vi "Transmitter HMI Main.vi"() -> ()   [LabVIEW 2025]
uses:
  Globals/Cancelled Global.vi
  Globals/Percent Complete Global.vi
  Globals/Light VISA Global.vi
  <vilib>/Instr/_visa.llb/VISA Configure Serial Port (Instr).vi
  Globals/Solenoid VISA Global.vi
  Globals/Touch VISA Global.vi
  Globals/Motor VISA Global.vi
  Globals/Wire VISA Global.vi
  Globals/QRCode VISA Global.vi
panel:
  in  "Enable Wire":bool
  in  "Enable Barcode":bool
  in  "Enable Motor":bool
  in  "Enable Light":bool
  in  "Enable Touch":bool
  in  "Enable Solenoid":bool
  in  "FREQUENCY CHANGER":bool
  in  "Barcode":bool
  in  "Wire":bool
  out "Start Transmission":bool
  out "Exit":bool
  out "Transmitting":bool
  out "Chosen Text":string
  out "Chosen Image Path":path caption="selected path"
  out "Chosen Transmission Method":u16(ring) items=["Barcode", "Wire", "Motor", "Touch", "Light", "Solenoid"]
  out "Chosen Data Type":u16(ring) items=["Text File", "Image File", "Image", "Text"]
  in  "Cancel Button":bool
  out "Transmission Progress:":dbl(slide) scale=0.0..100.0
  in  "Go":bool
  in  "Motor":bool
  in  "Touch":bool
  in  "Light":bool
  in  "Solenoid":bool
  in  "Image":bool
  in  "Text":bool
  # "TRANSMITTER"
  # "1: Select Data Type:"
  # "2: Select Method of Transmission:"
  # "3: BEGIN"
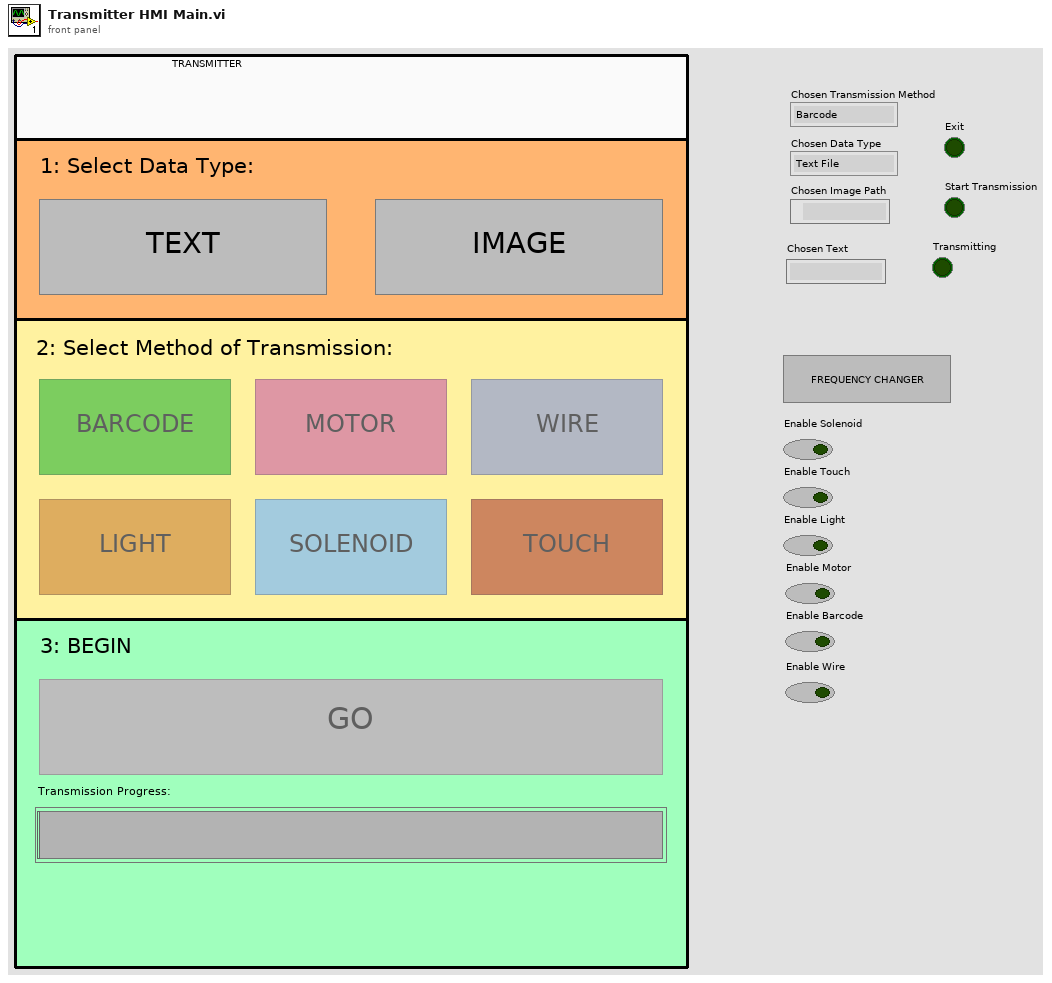
[diagram p1: front panel]
types:
  T1 = enum8{"Enabled", "Disabled", "Disabled and Grayed Out"}
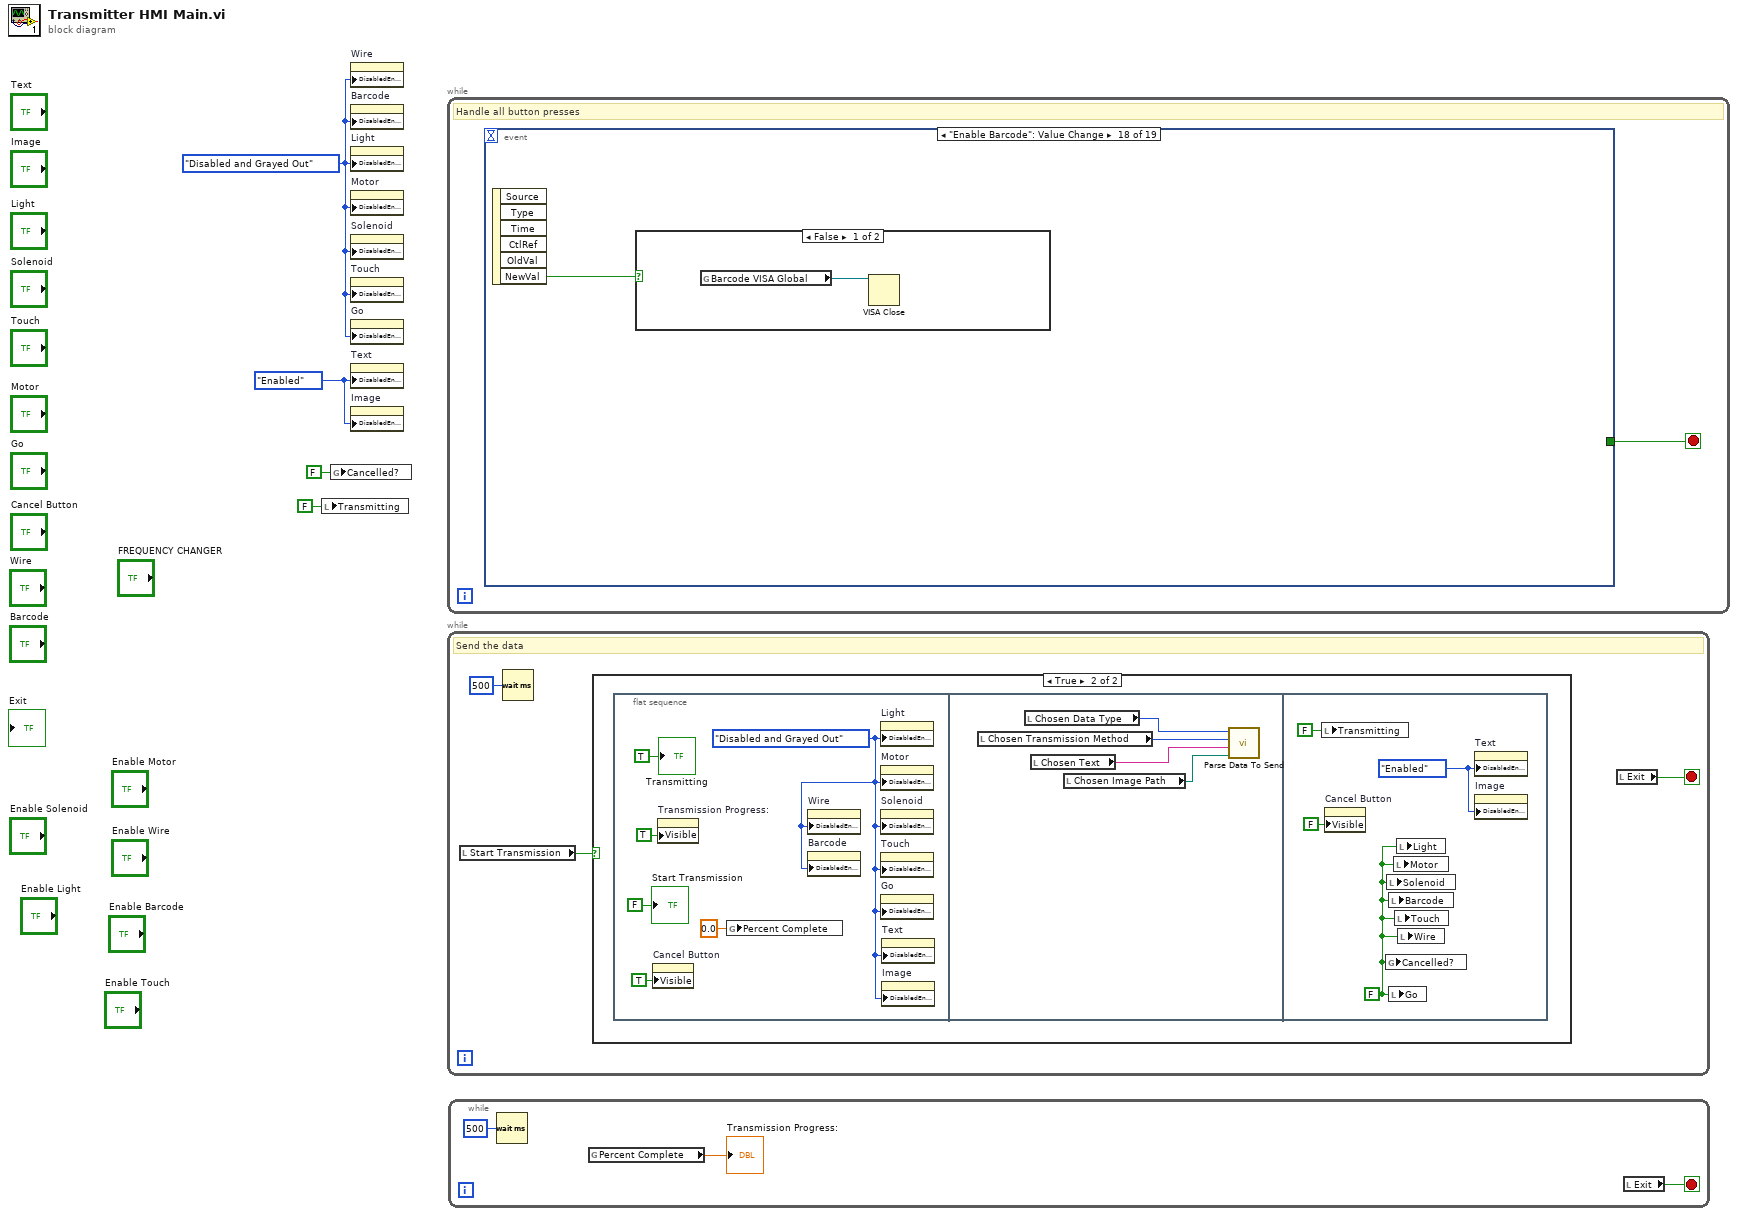
[diagram p0: block diagram]
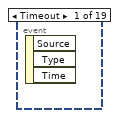
[diagram p3: hidden frame]
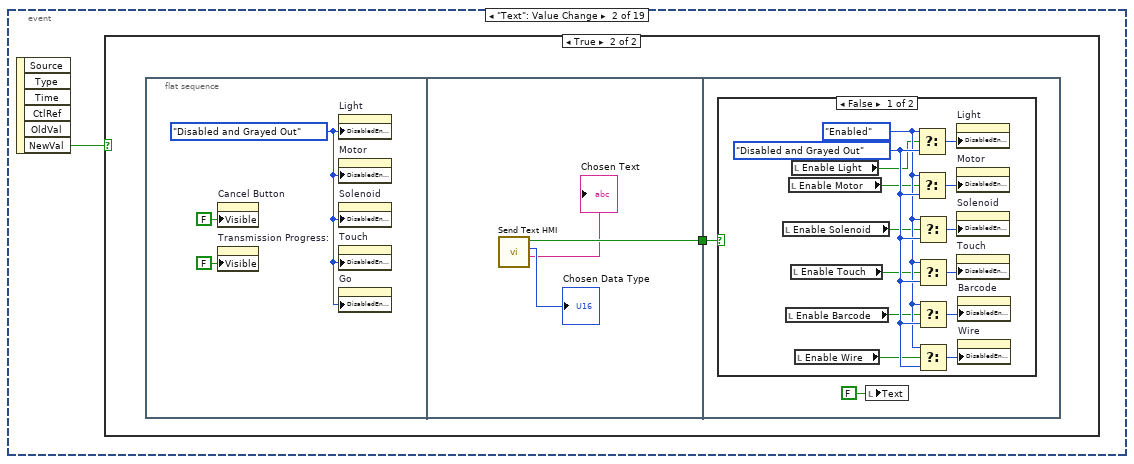
[diagram p4: hidden frame]
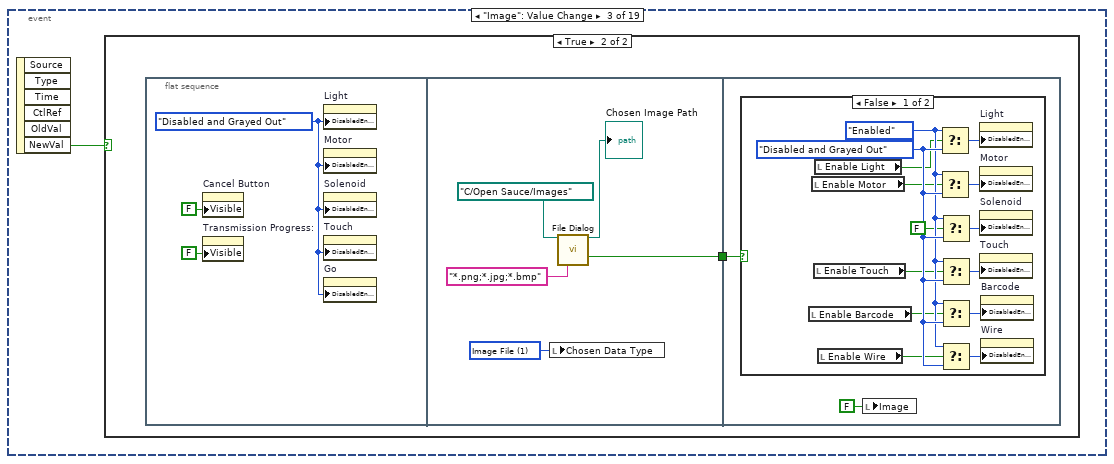
[diagram p7: hidden frame]
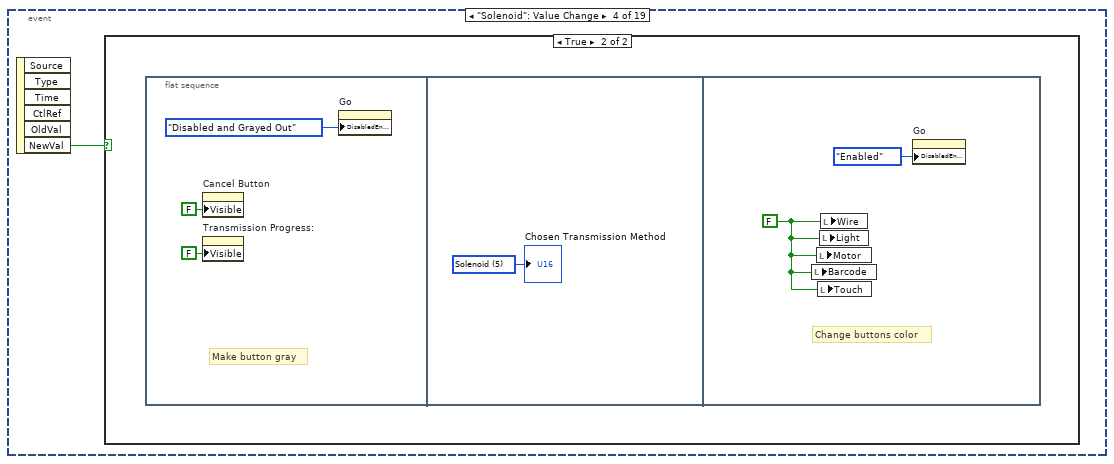
[diagram p10: hidden frame]
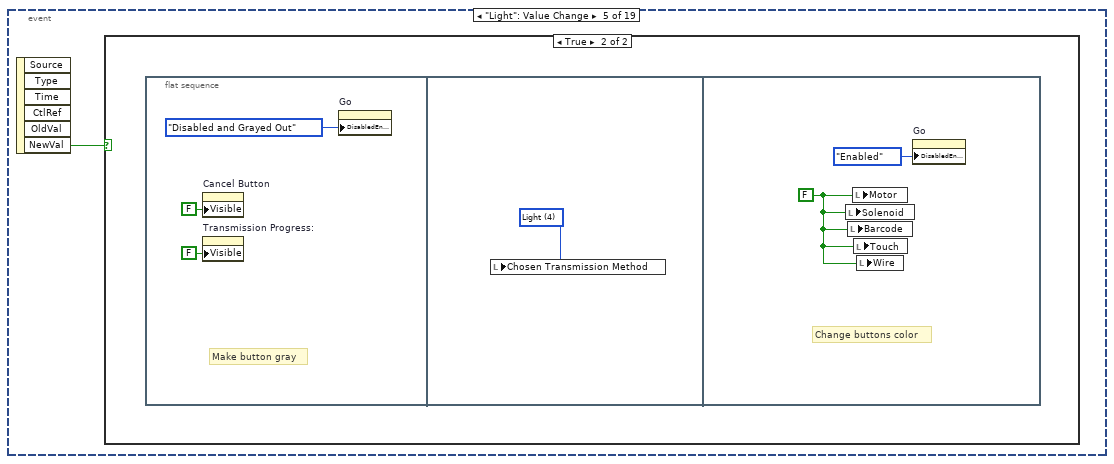
[diagram p12: hidden frame]
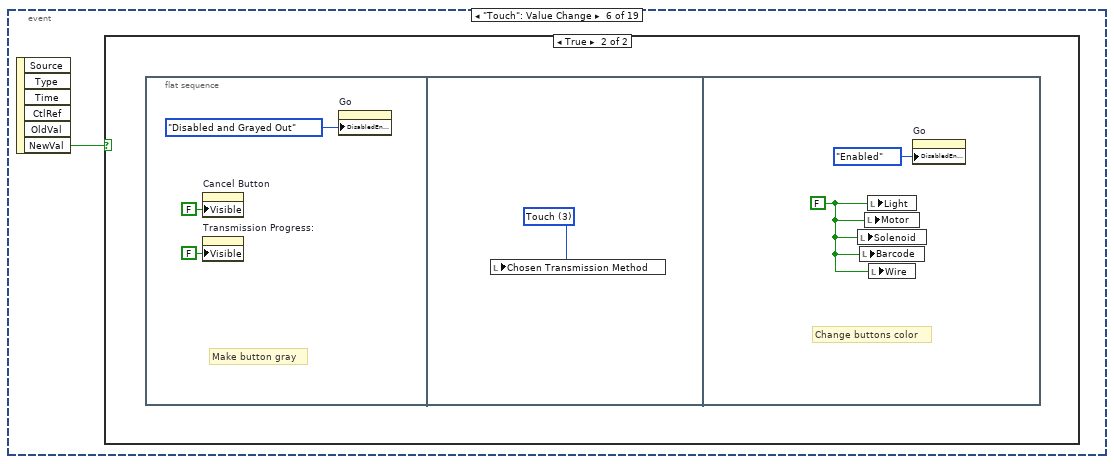
[diagram p14: hidden frame]
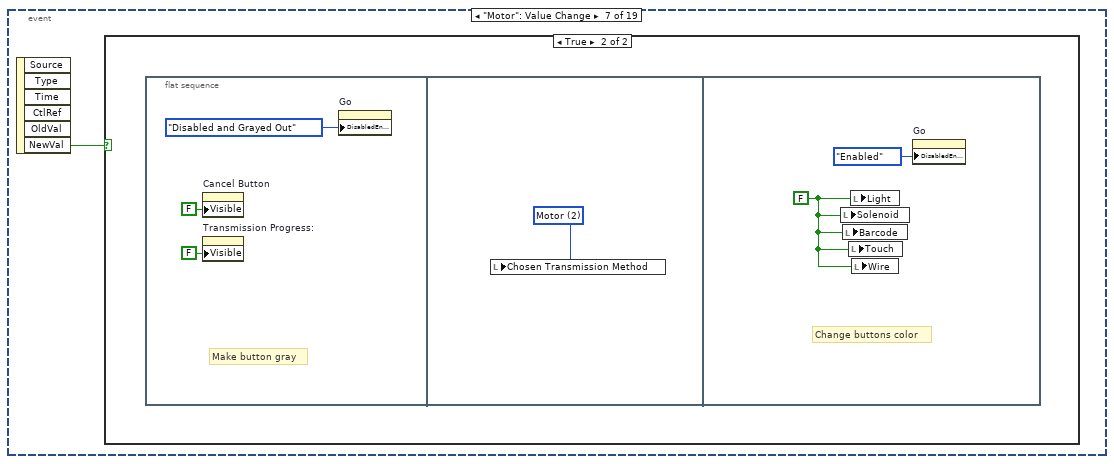
[diagram p16: hidden frame]
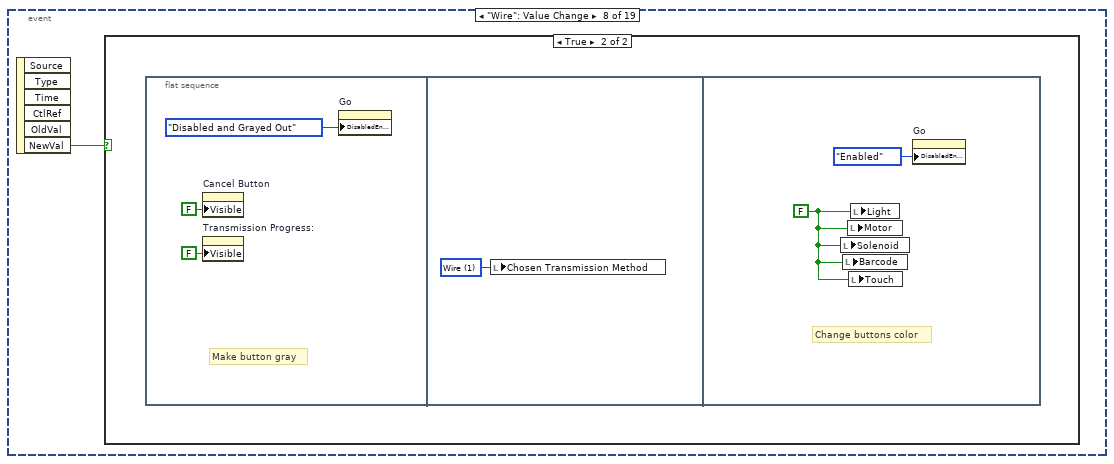
[diagram p18: hidden frame]
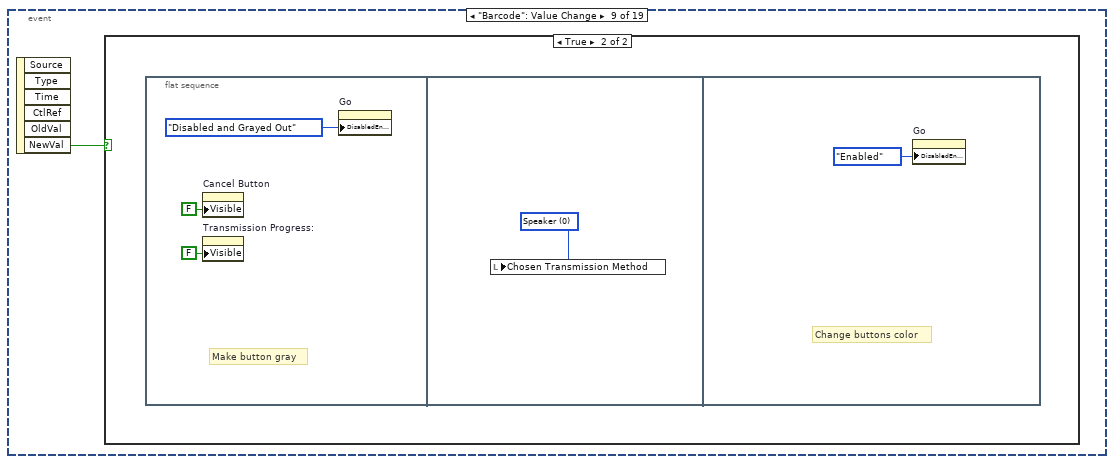
[diagram p20: hidden frame]
diagram:
  w2 = T1."Enabled" ("Disabled")
  w1 = T1."Disabled and Grayed Out" ("Disabled")
  n1 = local write "Transmitting"(FALSE ("Transmitting")) -> ()
  n2 = global write "Cancelled Global.vi" "Cancelled?"(FALSE ("Cancelled?")) -> ()
  n3 = property on="Wire" class="Bool (strict)"("DisabledEnum"=w1) -> ()  [unwired: 2 in, 2 out]
  n4 = property on="Barcode" class="Bool (strict)"("DisabledEnum"=w1) -> ()  [unwired: 2 in, 2 out]
  n5 = property on="Light" class="Bool (strict)"("DisabledEnum"=w1) -> ()  [unwired: 2 in, 2 out]
  n6 = property on="Motor" class="Bool (strict)"("DisabledEnum"=w1) -> ()  [unwired: 2 in, 2 out]
  n7 = property on="Solenoid" class="Bool (strict)"("DisabledEnum"=w1) -> ()  [unwired: 2 in, 2 out]
  n8 = property on="Touch" class="Bool (strict)"("DisabledEnum"=w1) -> ()  [unwired: 2 in, 2 out]
  n9 = property on="Go" class="Bool (strict)"("DisabledEnum"=w1) -> ()  [unwired: 2 in, 2 out]
  n10 = property on="Text" class="Bool (strict)"("DisabledEnum"=w2) -> ()  [unwired: 2 in, 2 out]
  n11 = property on="Image" class="Bool (strict)"("DisabledEnum"=w2) -> ()  [unwired: 2 in, 2 out]
  n12 = while {
    stop <- w5 stop-if-true
    # "Handle all button presses"
    n13 = event shown="[17] \"Enable Barcode\": Value Change" {
      selector: _ -> [_ _ _ _ _ _ _ _ _ _ _ _ _ _ _ _ _ _ _]
      dyn-events: _ -> [_ _ _ _ _ _ _ _ _ _ _ _ _ _ _ _ _ _ _]
      timeout: _ -> [_ _ _ _ _ _ _ _ _ _ _ _ _ _ _ _ _ _ _]
      tunnel: [_ _ _ _ _ _ _ _ _ TRUE _ _ _ _ _ _ _ _ _] -> w5
      event Timeout {
        n14 = event-data() -> ()  [unwired: 1 in, 3 out]
      }
      event "Text": Value Change {
        n15 = event-data() -> ("NewVal"=w6:bool)  [unwired: 1 in, 5 out]
        n16 = case shown="True" w6 {
          frame False {
          }
          frame True {
            n17 = flat-sequence {
              tunnel: [w13] -> w7
              tunnel: w7 -> [w15]
              frame #0 {
                w9 = T1."Disabled and Grayed Out" ("Disabled")
                n18 = property on="Cancel Button" class="Bool (strict)"("Visible"=FALSE) -> ()  [unwired: 2 in, 2 out]
                n19 = property on="Transmission Progress:" class="Slide (strict)"("Visible"=FALSE) -> ()  [unwired: 2 in, 2 out]
                n20 = property on="Light" class="Bool (strict)"("DisabledEnum"=w9) -> ()  [unwired: 2 in, 2 out]
                n21 = property on="Motor" class="Bool (strict)"("DisabledEnum"=w9) -> ()  [unwired: 2 in, 2 out]
                n22 = property on="Solenoid" class="Bool (strict)"("DisabledEnum"=w9) -> ()  [unwired: 2 in, 2 out]
                n23 = property on="Touch" class="Bool (strict)"("DisabledEnum"=w9) -> ()  [unwired: 2 in, 2 out]
                n24 = property on="Go" class="Bool (strict)"("DisabledEnum"=w9) -> ()  [unwired: 2 in, 2 out]
              }
              frame #1 {
                n25 = call "Send Text HMI.vi"() -> ("Chosen Text"=→"Chosen Text":string, "Chosen Data Type"=→"Chosen Data Type":u16, "Cancelled"=w13:bool)  [unwired: 9 in]
              }
              frame #2 {
                n26 = case shown="False" w15 {
                  frame False {
                    w23 = T1."Disabled and Grayed Out" ("Disabled")
                    w22 = T1."Enabled" ("Disabled")
                    n27 = local read "Enable Solenoid"() -> (w18:bool)
                    n28 = local read "Enable Barcode"() -> (w20:bool)
                    n29 = local read "Enable Motor"() -> (w17:bool)
                    n30 = local read "Enable Touch"() -> (w19:bool)
                    n31 = local read "Enable Light"() -> (w16:bool)
                    n32 = local read "Enable Wire"() -> (w21:bool)
                    n33 = Select(t=w22, s=w16, f=w23) -> (s? t:f=w29:T1)
                    n34 = Select(t=w22, s=w17, f=w23) -> (s? t:f=w28:T1)
                    n35 = Select(t=w22, s=w18, f=w23) -> (s? t:f=w27:T1)
                    n36 = Select(t=w22, s=w19, f=w23) -> (s? t:f=w26:T1)
                    n37 = Select(t=w22, s=w20, f=w23) -> (s? t:f=w25:T1)
                    n38 = Select(t=w22, s=w21, f=w23) -> (s? t:f=w24:T1)
                    n39 = property on="Light" class="Bool (strict)"("DisabledEnum"=w29) -> ()  [unwired: 2 in, 2 out]
                    n40 = property on="Motor" class="Bool (strict)"("DisabledEnum"=w28) -> ()  [unwired: 2 in, 2 out]
                    n41 = property on="Solenoid" class="Bool (strict)"("DisabledEnum"=w27) -> ()  [unwired: 2 in, 2 out]
                    n42 = property on="Touch" class="Bool (strict)"("DisabledEnum"=w26) -> ()  [unwired: 2 in, 2 out]
                    n43 = property on="Barcode" class="Bool (strict)"("DisabledEnum"=w25) -> ()  [unwired: 2 in, 2 out]
                    n44 = property on="Wire" class="Bool (strict)"("DisabledEnum"=w24) -> ()  [unwired: 2 in, 2 out]
                  }
                  frame True {
                  }
                }
                n45 = local write "Text"(FALSE ("Text")) -> ()
              }
            }
          }
        }
      }
      event "Image": Value Change {
        n46 = event-data() -> ("NewVal"=w30:bool)  [unwired: 1 in, 5 out]
        n47 = case shown="True" w30 {
          frame False {
          }
          frame True {
            n48 = flat-sequence {
              tunnel: [w37] -> w31
              tunnel: w31 -> [w40]
              frame #0 {
                w33 = T1."Disabled and Grayed Out" ("Disabled")
                n49 = property on="Cancel Button" class="Bool (strict)"("Visible"=FALSE) -> ()  [unwired: 2 in, 2 out]
                n50 = property on="Transmission Progress:" class="Slide (strict)"("Visible"=FALSE) -> ()  [unwired: 2 in, 2 out]
                n51 = property on="Light" class="Bool (strict)"("DisabledEnum"=w33) -> ()  [unwired: 2 in, 2 out]
                n52 = property on="Motor" class="Bool (strict)"("DisabledEnum"=w33) -> ()  [unwired: 2 in, 2 out]
                n53 = property on="Solenoid" class="Bool (strict)"("DisabledEnum"=w33) -> ()  [unwired: 2 in, 2 out]
                n54 = property on="Touch" class="Bool (strict)"("DisabledEnum"=w33) -> ()  [unwired: 2 in, 2 out]
                n55 = property on="Go" class="Bool (strict)"("DisabledEnum"=w33) -> ()  [unwired: 2 in, 2 out]
              }
              frame #1 {
                w35 = u16 1 items=["Text File", "Image File", "Image", "Text"] ("Chosen Data Type")
                n56 = local write "Chosen Data Type"(w35) -> ()
                n57 = call "File Dialog"("start path"=path "C:/Open Sauce/Images", "pattern (all files)"="*.png;*.jpg;*.bmp") -> ("selected path"=→"Chosen Image Path":path, "cancelled"=w37:bool)  [unwired: 10 in, 2 out]
              }
              frame #2 {
                n58 = case shown="False" w40 {
                  frame False {
                    w49 = T1."Disabled and Grayed Out" ("Disabled")
                    w48 = T1."Enabled" ("Disabled")
                    n59 = local read "Enable Barcode"() -> (w46:bool)
                    n60 = local read "Enable Motor"() -> (w44:bool)
                    n61 = local read "Enable Touch"() -> (w45:bool)
                    n62 = local read "Enable Light"() -> (w43:bool)
                    n63 = local read "Enable Wire"() -> (w47:bool)
                    n64 = Select(t=w48, s=w43, f=w49) -> (s? t:f=w55:T1)
                    n65 = Select(t=w48, s=w44, f=w49) -> (s? t:f=w54:T1)
                    n66 = Select(t=w48, s=FALSE, f=w49) -> (s? t:f=w53:T1)
                    n67 = Select(t=w48, s=w45, f=w49) -> (s? t:f=w52:T1)
                    n68 = Select(t=w48, s=w46, f=w49) -> (s? t:f=w51:T1)
                    n69 = Select(t=w48, s=w47, f=w49) -> (s? t:f=w50:T1)
                    n70 = property on="Light" class="Bool (strict)"("DisabledEnum"=w55) -> ()  [unwired: 2 in, 2 out]
                    n71 = property on="Motor" class="Bool (strict)"("DisabledEnum"=w54) -> ()  [unwired: 2 in, 2 out]
                    n72 = property on="Solenoid" class="Bool (strict)"("DisabledEnum"=w53) -> ()  [unwired: 2 in, 2 out]
                    n73 = property on="Touch" class="Bool (strict)"("DisabledEnum"=w52) -> ()  [unwired: 2 in, 2 out]
                    n74 = property on="Barcode" class="Bool (strict)"("DisabledEnum"=w51) -> ()  [unwired: 2 in, 2 out]
                    n75 = property on="Wire" class="Bool (strict)"("DisabledEnum"=w50) -> ()  [unwired: 2 in, 2 out]
                  }
                  frame True {
                  }
                }
                n76 = local write "Image"(FALSE ("Text")) -> ()
              }
            }
          }
        }
      }
      event "Solenoid": Value Change {
        n77 = event-data() -> ("NewVal"=w56:bool)  [unwired: 1 in, 5 out]
        n78 = case shown="True" w56 {
          frame False {
          }
          frame True {
            n79 = flat-sequence {
              frame #0 {
                # "Make button gray"
                n80 = property on="Cancel Button" class="Bool (strict)"("Visible"=FALSE) -> ()  [unwired: 2 in, 2 out]
                n81 = property on="Transmission Progress:" class="Slide (strict)"("Visible"=FALSE) -> ()  [unwired: 2 in, 2 out]
                n82 = property on="Go" class="Bool (strict)"("DisabledEnum"=T1."Disabled and Grayed Out" ("Disabled")) -> ()  [unwired: 2 in, 2 out]
              }
              frame #1 {
                w60 = u16 5 items=["Speaker", "Wire", "Motor", "Touch", "Light", "Solenoid"] ("Chosen Transmission Method")
                "Chosen Transmission Method" <- w60
              }
              frame #2 {
                w61 = FALSE ("Text")
                # "Change buttons color"
                n83 = local write "Barcode"(w61) -> ()
                n84 = local write "Motor"(w61) -> ()
                n85 = local write "Touch"(w61) -> ()
                n86 = local write "Light"(w61) -> ()
                n87 = local write "Wire"(w61) -> ()
                n88 = property on="Go" class="Bool (strict)"("DisabledEnum"=T1."Enabled" ("Disabled")) -> ()  [unwired: 2 in, 2 out]
              }
            }
          }
        }
      }
      event "Light": Value Change {
        n89 = event-data() -> ("NewVal"=w63:bool)  [unwired: 1 in, 5 out]
        n90 = case shown="True" w63 {
          frame False {
          }
          frame True {
            n91 = flat-sequence {
              frame #0 {
                # "Make button gray"
                n92 = property on="Cancel Button" class="Bool (strict)"("Visible"=FALSE) -> ()  [unwired: 2 in, 2 out]
                n93 = property on="Transmission Progress:" class="Slide (strict)"("Visible"=FALSE) -> ()  [unwired: 2 in, 2 out]
                n94 = property on="Go" class="Bool (strict)"("DisabledEnum"=T1."Disabled and Grayed Out" ("Disabled")) -> ()  [unwired: 2 in, 2 out]
              }
              frame #1 {
                w67 = u16 4 items=["Speaker", "Wire", "Motor", "Touch", "Light", "Solenoid"] ("Chosen Transmission Method")
                n95 = local write "Chosen Transmission Method"(w67) -> ()
              }
              frame #2 {
                w68 = FALSE ("Text")
                # "Change buttons color"
                n96 = local write "Solenoid"(w68) -> ()
                n97 = local write "Barcode"(w68) -> ()
                n98 = local write "Motor"(w68) -> ()
                n99 = local write "Touch"(w68) -> ()
                n100 = local write "Wire"(w68) -> ()
                n101 = property on="Go" class="Bool (strict)"("DisabledEnum"=T1."Enabled" ("Disabled")) -> ()  [unwired: 2 in, 2 out]
              }
            }
          }
        }
      }
      event "Touch": Value Change {
        n102 = event-data() -> ("NewVal"=w70:bool)  [unwired: 1 in, 5 out]
        n103 = case shown="True" w70 {
          frame False {
          }
          frame True {
            n104 = flat-sequence {
              frame #0 {
                # "Make button gray"
                n105 = property on="Cancel Button" class="Bool (strict)"("Visible"=FALSE) -> ()  [unwired: 2 in, 2 out]
                n106 = property on="Transmission Progress:" class="Slide (strict)"("Visible"=FALSE) -> ()  [unwired: 2 in, 2 out]
                n107 = property on="Go" class="Bool (strict)"("DisabledEnum"=T1."Disabled and Grayed Out" ("Disabled")) -> ()  [unwired: 2 in, 2 out]
              }
              frame #1 {
                w74 = u16 3 items=["Speaker", "Wire", "Motor", "Touch", "Light", "Solenoid"] ("Chosen Transmission Method")
                n108 = local write "Chosen Transmission Method"(w74) -> ()
              }
              frame #2 {
                w75 = FALSE ("Text")
                # "Change buttons color"
                n109 = local write "Solenoid"(w75) -> ()
                n110 = local write "Barcode"(w75) -> ()
                n111 = local write "Motor"(w75) -> ()
                n112 = local write "Light"(w75) -> ()
                n113 = local write "Wire"(w75) -> ()
                n114 = property on="Go" class="Bool (strict)"("DisabledEnum"=T1."Enabled" ("Disabled")) -> ()  [unwired: 2 in, 2 out]
              }
            }
          }
        }
      }
      event "Motor": Value Change {
        n115 = event-data() -> ("NewVal"=w77:bool)  [unwired: 1 in, 5 out]
        n116 = case shown="True" w77 {
          frame False {
          }
          frame True {
            n117 = flat-sequence {
              frame #0 {
                # "Make button gray"
                n118 = property on="Cancel Button" class="Bool (strict)"("Visible"=FALSE) -> ()  [unwired: 2 in, 2 out]
                n119 = property on="Transmission Progress:" class="Slide (strict)"("Visible"=FALSE) -> ()  [unwired: 2 in, 2 out]
                n120 = property on="Go" class="Bool (strict)"("DisabledEnum"=T1."Disabled and Grayed Out" ("Disabled")) -> ()  [unwired: 2 in, 2 out]
              }
              frame #1 {
                w81 = u16 2 items=["Speaker", "Wire", "Motor", "Touch", "Light", "Solenoid"] ("Chosen Transmission Method")
                n121 = local write "Chosen Transmission Method"(w81) -> ()
              }
              frame #2 {
                w82 = FALSE ("Text")
                # "Change buttons color"
                n122 = local write "Solenoid"(w82) -> ()
                n123 = local write "Barcode"(w82) -> ()
                n124 = local write "Touch"(w82) -> ()
                n125 = local write "Light"(w82) -> ()
                n126 = local write "Wire"(w82) -> ()
                n127 = property on="Go" class="Bool (strict)"("DisabledEnum"=T1."Enabled" ("Disabled")) -> ()  [unwired: 2 in, 2 out]
              }
            }
          }
        }
      }
      event "Wire": Value Change {
        n128 = event-data() -> ("NewVal"=w84:bool)  [unwired: 1 in, 5 out]
        n129 = case shown="True" w84 {
          frame False {
          }
          frame True {
            n130 = flat-sequence {
              frame #0 {
                # "Make button gray"
                n131 = property on="Cancel Button" class="Bool (strict)"("Visible"=FALSE) -> ()  [unwired: 2 in, 2 out]
                n132 = property on="Transmission Progress:" class="Slide (strict)"("Visible"=FALSE) -> ()  [unwired: 2 in, 2 out]
                n133 = property on="Go" class="Bool (strict)"("DisabledEnum"=T1."Disabled and Grayed Out" ("Disabled")) -> ()  [unwired: 2 in, 2 out]
              }
              frame #1 {
                w88 = u16 1 items=["Speaker", "Wire", "Motor", "Touch", "Light", "Solenoid"] ("Chosen Transmission Method")
                n134 = local write "Chosen Transmission Method"(w88) -> ()
              }
              frame #2 {
                w89 = FALSE ("Text")
                # "Change buttons color"
                n135 = local write "Solenoid"(w89) -> ()
                n136 = local write "Barcode"(w89) -> ()
                n137 = local write "Motor"(w89) -> ()
                n138 = local write "Touch"(w89) -> ()
                n139 = local write "Light"(w89) -> ()
                n140 = property on="Go" class="Bool (strict)"("DisabledEnum"=T1."Enabled" ("Disabled")) -> ()  [unwired: 2 in, 2 out]
              }
            }
          }
        }
      }
      event "Barcode": Value Change {
        n141 = event-data() -> ("NewVal"=w91:bool)  [unwired: 1 in, 5 out]
        n142 = case shown="True" w91 {
          frame False {
          }
          frame True {
            n143 = flat-sequence {
              frame #0 {
                # "Make button gray"
                n144 = property on="Cancel Button" class="Bool (strict)"("Visible"=FALSE) -> ()  [unwired: 2 in, 2 out]
                n145 = property on="Transmission Progress:" class="Slide (strict)"("Visible"=FALSE) -> ()  [unwired: 2 in, 2 out]
                n146 = property on="Go" class="Bool (strict)"("DisabledEnum"=T1."Disabled and Grayed Out" ("Disabled")) -> ()  [unwired: 2 in, 2 out]
              }
              frame #1 {
                w95 = u16 0 items=["Speaker", "Wire", "Motor", "Touch", "Light", "Solenoid"] ("Chosen Transmission Method")
                n147 = local write "Chosen Transmission Method"(w95) -> ()
              }
              frame #2 {
                # "Change buttons color"
                n148 = property on="Go" class="Bool (strict)"("DisabledEnum"=T1."Enabled" ("Disabled")) -> ()  [unwired: 2 in, 2 out]
              }
            }
          }
        }
      }
      event Panel Close {
        n149 = event-data() -> ()  [unwired: 1 in, 4 out]
      }
      event "Go": Value Change {
        n150 = event-data() -> ("NewVal"=w98:bool)  [unwired: 1 in, 5 out]
        n151 = case shown="True" w98 {
          frame False {
          }
          frame True {
            n152 = local write "Cancel Button"(FALSE ("Cancel Button")) -> ()
            n153 = local write "Start Transmission"(TRUE ("Start Transmission")) -> ()
          }
        }
      }
      event "Cancel Button": Value Change {
        n154 = event-data() -> ("NewVal"=w101:bool)  [unwired: 1 in, 5 out]
        n155 = global write "Cancelled Global.vi" "Cancelled?"(w101) -> ()
      }
      event "FREQUENCY CHANGER": Value Change {
        n156 = event-data() -> ("NewVal"=w102:bool)  [unwired: 1 in, 5 out]
        n157 = case shown="True" w102 {
          frame False {
          }
          frame True {
            n158 = call "Frequency Changer.vi"() -> ()  [unwired: 12 in]
            n159 = local write "FREQUENCY CHANGER"(FALSE ("FREQUENCY CHANGER")) -> ()
          }
        }
      }
      event "Enable Solenoid": Value Change {
        n160 = event-data() -> ("NewVal"=w104:bool)  [unwired: 1 in, 5 out]
        n161 = case shown="False" w104 {
          frame False {
            n162 = global read "Solenoid VISA Global.vi" "Solenoid VISA Global"() -> (w105:refnum<visa-resource-name>)
            n163 = VISA Close(VISA resource name=w105) -> ()  [unwired: 1 in, 1 out]
          }
          frame True {
            n164 = call-poly "VISA Configure Serial Port"("VISA resource name"=refnum<visa-resource-name> "SOLENOID_TRANSMITTER") -> ("VISA resource name out"=w106:refnum<visa-resource-name>)  [unwired: 13 in, 1 out]
            n165 = global write "Solenoid VISA Global.vi" "Solenoid VISA Global"(w106) -> ()
          }
        }
      }
      event "Enable Touch": Value Change {
        n166 = event-data() -> ("NewVal"=w108:bool)  [unwired: 1 in, 5 out]
        n167 = case shown="True" w108 {
          frame False {
            n168 = global read "Touch VISA Global.vi" "Touch VISA Global"() -> (w109:refnum<visa-resource-name>)
            n169 = VISA Close(VISA resource name=w109) -> ()  [unwired: 1 in, 1 out]
          }
          frame True {
            n170 = call-poly "VISA Configure Serial Port"("VISA resource name"=refnum<visa-resource-name> "TOUCH_TRANSMITTER") -> ("VISA resource name out"=w110:refnum<visa-resource-name>)  [unwired: 13 in, 1 out]
            n171 = global write "Touch VISA Global.vi" "Touch VISA Global"(w110) -> ()
          }
        }
      }
      event "Enable Light": Value Change {
        n172 = event-data() -> ("NewVal"=w112:bool)  [unwired: 1 in, 5 out]
        n173 = case shown="True" w112 {
          frame False {
            n174 = global read "Touch VISA Global.vi" "Touch VISA Global"() -> (w113:refnum<visa-resource-name>)
            n175 = VISA Close(VISA resource name=w113) -> ()  [unwired: 1 in, 1 out]
          }
          frame True {
            n176 = call-poly "VISA Configure Serial Port"("VISA resource name"=refnum<visa-resource-name> "LIGHT_TRANSMITTER") -> ("VISA resource name out"=w115:refnum<visa-resource-name>)  [unwired: 13 in, 1 out]
            n177 = global write "Light VISA Global.vi" "LIGHT VISA resource name out"(w115) -> ()
          }
        }
      }
      event "Enable Motor": Value Change {
        n178 = event-data() -> ("NewVal"=w116:bool)  [unwired: 1 in, 5 out]
        n179 = case shown="True" w116 {
          frame False {
            n180 = global read "Motor VISA Global.vi" "Motor VISA Global"() -> (w117:refnum<visa-resource-name>)
            n181 = VISA Close(VISA resource name=w117) -> ()  [unwired: 1 in, 1 out]
          }
          frame True {
            n182 = call-poly "VISA Configure Serial Port"("VISA resource name"=refnum<visa-resource-name> "MOTOR_TRANSMITTER") -> ("VISA resource name out"=w118:refnum<visa-resource-name>)  [unwired: 13 in, 1 out]
            n183 = global write "Motor VISA Global.vi" "Motor VISA Global"(w118) -> ()
          }
        }
      }
      event "Enable Barcode": Value Change {
        n184 = event-data() -> ("NewVal"=w120:bool)  [unwired: 1 in, 5 out]
        n185 = case shown="False" w120 {
          frame False {
            n186 = global read "QRCode VISA Global.vi" "Barcode VISA Global"() -> (w121:refnum<visa-resource-name>)
            n187 = VISA Close(VISA resource name=w121) -> ()  [unwired: 1 in, 1 out]
          }
          frame True {
            n188 = call-poly "VISA Configure Serial Port"("VISA resource name"=refnum<visa-resource-name> "BARCODE_TRANSMITTER") -> ("VISA resource name out"=w122:refnum<visa-resource-name>)  [unwired: 13 in, 1 out]
            n189 = global write "QRCode VISA Global.vi" "Barcode VISA Global"(w122) -> ()
          }
        }
      }
      event "Enable Wire": Value Change {
        n190 = event-data() -> ("NewVal"=w124:bool)  [unwired: 1 in, 5 out]
        n191 = case shown="True" w124 {
          frame False {
            n192 = global read "Wire VISA Global.vi" "Wire VISA Global"() -> (w125:refnum<visa-resource-name>)
            n193 = VISA Close(VISA resource name=w125) -> ()  [unwired: 1 in, 1 out]
          }
          frame True {
            n194 = call-poly "VISA Configure Serial Port"("VISA resource name"=refnum<visa-resource-name> "WIRE_TRANSMITTER", "baud rate (9600)"=u32 57600) -> ("VISA resource name out"=w127:refnum<visa-resource-name>)  [unwired: 12 in, 1 out]
            n195 = global write "Wire VISA Global.vi" "Wire VISA Global"(w127) -> ()
          }
        }
      }
    }
  }
  n196 = while {
    stop <- w131 stop-if-true
    # "Send the data"
    n197 = local read "Start Transmission"() -> (w130:bool)
    n198 = Wait (ms)(milliseconds to wait=u32 500) -> ()  [unwired: 1 out]
    n199 = case shown="True" w130 {
      frame False {
      }
      frame True {
        n200 = flat-sequence {
          frame #0 {
            w132 = T1."Disabled and Grayed Out" ("Disabled")
            n201 = property on="Cancel Button" class="Bool (strict)"("Visible"=TRUE) -> ()  [unwired: 2 in, 2 out]
            n202 = property on="Transmission Progress:" class="Slide (strict)"("Visible"=TRUE) -> ()  [unwired: 2 in, 2 out]
            n203 = global write "Percent Complete Global.vi" "Percent Complete"(0.0 ("Percent Complete")) -> ()
            n204 = property on="Wire" class="Bool (strict)"("DisabledEnum"=w132) -> ()  [unwired: 2 in, 2 out]
            n205 = property on="Barcode" class="Bool (strict)"("DisabledEnum"=w132) -> ()  [unwired: 2 in, 2 out]
            n206 = property on="Light" class="Bool (strict)"("DisabledEnum"=w132) -> ()  [unwired: 2 in, 2 out]
            n207 = property on="Motor" class="Bool (strict)"("DisabledEnum"=w132) -> ()  [unwired: 2 in, 2 out]
            n208 = property on="Solenoid" class="Bool (strict)"("DisabledEnum"=w132) -> ()  [unwired: 2 in, 2 out]
            n209 = property on="Touch" class="Bool (strict)"("DisabledEnum"=w132) -> ()  [unwired: 2 in, 2 out]
            n210 = property on="Go" class="Bool (strict)"("DisabledEnum"=w132) -> ()  [unwired: 2 in, 2 out]
            n211 = property on="Text" class="Bool (strict)"("DisabledEnum"=w132) -> ()  [unwired: 2 in, 2 out]
            n212 = property on="Image" class="Bool (strict)"("DisabledEnum"=w132) -> ()  [unwired: 2 in, 2 out]
            "Start Transmission" <- FALSE ("Start Transmission")
            "Transmitting" <- TRUE ("Transmitting")
          }
          frame #1 {
            n213 = local read "Chosen Transmission Method"() -> (w139:u16)
            n214 = local read "Chosen Data Type"() -> (w138:u16)
            n215 = local read "Chosen Text"() -> (w140:string)
            n216 = local read "Chosen Image Path"() -> (w141:path)
            n217 = call "Parse Data To Send.vi"("Chosen Image Path"=w141, "Chosen Text"=w140, "Chosen Transmission Method"=w139, "Chosen Data Type"=w138) -> ()  [unwired: 8 in]
          }
          frame #2 {
            w142 = FALSE ("Go")
            w143 = T1."Enabled" ("Disabled")
            n218 = local write "Transmitting"(FALSE ("Transmitting")) -> ()
            n219 = property on="Cancel Button" class="Bool (strict)"("Visible"=FALSE) -> ()  [unwired: 2 in, 2 out]
            n220 = global write "Cancelled Global.vi" "Cancelled?"(w142) -> ()
            n221 = local write "Solenoid"(w142) -> ()
            n222 = local write "Barcode"(w142) -> ()
            n223 = local write "Go"(w142) -> ()
            n224 = local write "Motor"(w142) -> ()
            n225 = local write "Touch"(w142) -> ()
            n226 = local write "Light"(w142) -> ()
            n227 = local write "Wire"(w142) -> ()
            n228 = property on="Text" class="Bool (strict)"("DisabledEnum"=w143) -> ()  [unwired: 2 in, 2 out]
            n229 = property on="Image" class="Bool (strict)"("DisabledEnum"=w143) -> ()  [unwired: 2 in, 2 out]
          }
        }
      }
    }
    n230 = local read "Exit"() -> (w131:bool)
  }
  n231 = while {
    stop <- w148 stop-if-true
    n232 = Wait (ms)(milliseconds to wait=u32 500) -> ()  [unwired: 1 out]
    n233 = global read "Percent Complete Global.vi" "Percent Complete"() -> (→"Transmission Progress:":dbl)
    n234 = local read "Exit"() -> (w148:bool)
  }
